vi "A_Leaglag_subVi.vi"(6 "LL x":dbl, 7 "Pole":dbl=-2.4, 9 "Zero":dbl=-1000000000000.0, 10 "LL x_prev":dbl, 11 "LL y_prev":dbl) -> (1 "y*inv_gain":dbl, 2 "LL x out":dbl, 3 "LL y":dbl)   [LabVIEW 2011]
panel:
  out "inv_gain":dbl
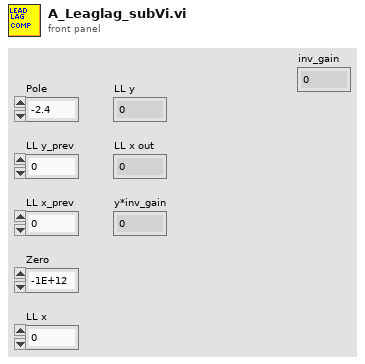
[diagram p1: front panel]
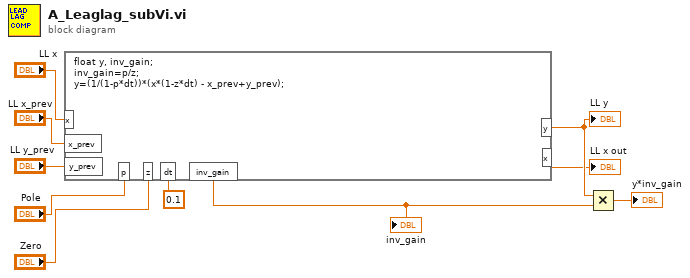
[diagram p0: block diagram]
diagram:
  n1 = formula code="float y, inv_gain;\ninv_gain=p/z;\ny=(1/(1-p*dt))*(x*(1-z*dt) - x_prev+y_prev);"("x"="LL x", "x_prev"="LL x_prev", "y_prev"="LL y_prev", "p"="Pole", "z"="Zero", "dt"=0.1 ("input variable")) -> ("y"=w8:dbl, "inv_gain"=w7:dbl, "x"=→"LL x out":dbl)
  "LL y" <- w8
  "inv_gain" <- w7
  n2 = Multiply(x=w8, y=w7) -> (x*y=→"y*inv_gain":dbl)
